vi "Get Remote Terminal Endpoint.vi"(8 "error in":errorcluster, 9 "direction":T1, 11 "message in":T4 format="%.0x") -> (0 "error out":errorcluster, 2 "remote terminal":T2, 3 "message out":T4 format="%.0x", 4 "found?":bool)   [LabVIEW 2020, in "AIM MIL-STD-1553 Scripting.lvlib"]
uses:
  AIM MIL-STD-1553 Scripting.lvlib
  <vilib>/NI VeriStand/Custom Device API/Custom Device Item Ref.ctl
  Shared/Terminal Endpoint.ctl
  Shared/Address.ctl
  Shared/Direction.ctl
  Constants.vi
  <vilib>/NI VeriStand/Custom Device API/Get Item Property (U16).vi
  <vilib>/NI VeriStand/Custom Device API/Custom Device API.lvlib
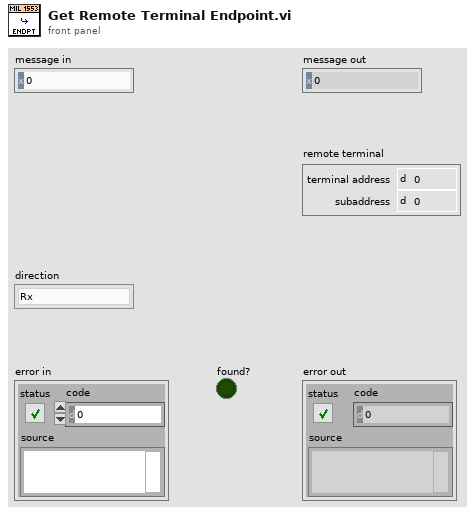
[diagram p1: front panel]
types:
  T1 = typedef "Direction.ctl" = enum16{"Rx", "Tx"}
  T2 = typedef "Terminal Endpoint.ctl" = cluster{"terminal address":T3, "subaddress":T3}
  T3 = typedef "Address.ctl" = u16
  T4 = typedef "Custom Device API.lvlib/Custom Device Item Ref.ctl" = u64
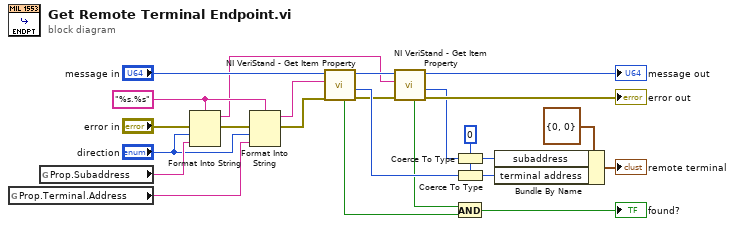
[diagram p0: block diagram]
diagram:
  w12 = "%s.%s" ("format string")
  w14 = T3 0 ("terminal address")
  n1 = global read "Constants.vi" "Prop.Terminal.Address"() -> (w8:string)
  n2 = global read "Constants.vi" "Prop.Subaddress"() -> (w11:string)
  n3 = Format Into String(format string=w12, error in="error in", "direction", w11) -> (resulting string=w10:string, error out=w2:errorcluster)  [unwired: 1 in]
  n4 = Format Into String(format string=w12, error in=w2, "direction", w8) -> (resulting string=w13:string, error out=w1:errorcluster)  [unwired: 1 in]
  n5 = call-poly <vilib>:"NI VeriStand - Get Item Property.vi"("error in (no error)"=w1, "Property Name"=w13, "Item Ref in"="message in") -> ("error out"=w4:errorcluster, "Value"=w16:u16, "Item Ref out"=w23:T4, "Found?"=w7:bool)  [unwired: 5 in]
  n6 = call-poly <vilib>:"NI VeriStand - Get Item Property.vi"("error in (no error)"=w4, "Property Name"=w10, "Item Ref in"=w23) -> ("error out"=→"error out":errorcluster, "Value"=w15:u16, "Item Ref out"=→"message out":T4, "Found?"=w6:bool)  [unwired: 5 in]
  n7 = Coerce To Type(0:w15, 1:w14) -> (2:w20:T3)
  n8 = Coerce To Type(0:w16, 1:w14) -> (2:w19:T3)
  n9 = And(x=w6, y=w7) -> (x .and. y?=→"found?":bool)
  n10 = Bundle By Name(cluster=T2 {"terminal address"=0, "subaddress"=0} ("remote terminal"), "subaddress"=w20, "terminal address"=w19) -> (→"remote terminal":T2)
